vi "Comparator_Dots_Coordinates-1.vi"(0 "X1":dbl, 5 "Y1":dbl, 7 "(X+dX)1":dbl, 9 "(Y+dY)1":dbl, 11 "X2":dbl, 12 "Y2":dbl, 13 "(X+dX)2":dbl, 14 "(Y+dY)2":dbl) -> (4 "X1=X2,Y1=Y2 (1)":bool, 8 "X1(2)=X2(2),Y1(2)=Y2(2) (2)":bool, 15 "(1) OR (2) = (3)":bool)   [LabVIEW 2017]
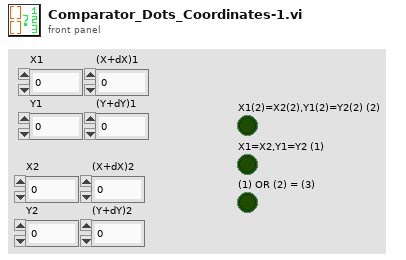
[diagram p1: front panel]
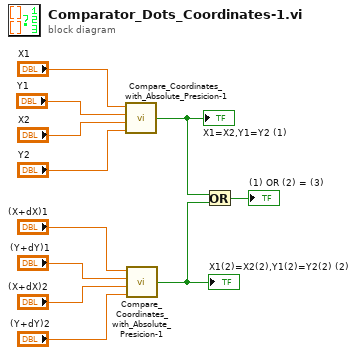
[diagram p0: block diagram]
diagram:
  n1 = call "Compare_Coordinates_with_Absolute_Presicion-1.vi"("X 1"="X1", "Y 1"="Y1", "X 2"="X2", "Y 2"="Y2") -> ("[OUT] Same coordinates?"=w9:bool)  [unwired: 1 in]
  "X1=X2,Y1=Y2 (1)" <- w9
  n2 = call "Compare_Coordinates_with_Absolute_Presicion-1.vi"("X 1"="(X+dX)1", "Y 1"="(Y+dY)1", "X 2"="(X+dX)2", "Y 2"="(Y+dY)2") -> ("[OUT] Same coordinates?"=w4:bool)  [unwired: 1 in]
  "X1(2)=X2(2),Y1(2)=Y2(2) (2)" <- w4
  n3 = Or(x=w9, y=w4) -> (x .or. y?=→"(1) OR (2) = (3)":bool)
